vi "GOOP_VI_Provider_Interface.vi"() -> (3 "Interface Table":T1)   [LabVIEW 2014]
uses:
  <resource>/Framework/Providers/API/Provider_Interface.ctl
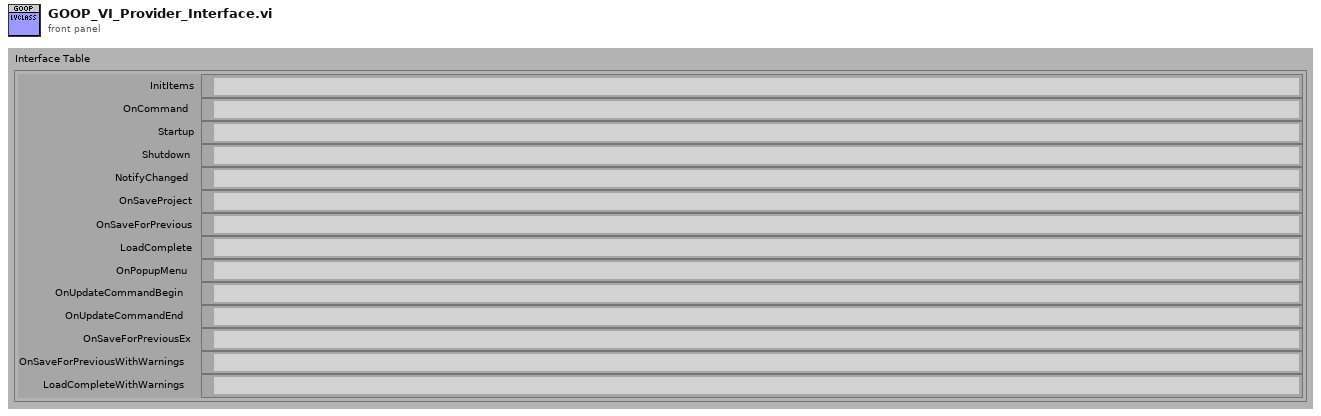
[diagram p1: front panel]
types:
  T1 = typedef "Provider_Interface.ctl" = cluster{"InitItems":path, "OnCommand":path, "Startup":path, "Shutdown":path, "NotifyChanged":path, "OnSaveProject":path, "OnSaveForPrevious":path, "LoadComplete":path, "OnPopupMenu":path, "OnUpdateCommandBegin":path, "OnUpdateCommandEnd":path, "OnSaveForPreviousEx":path, "OnSaveForPreviousWithWarnings":path, "LoadCompleteWithWarnings":path}
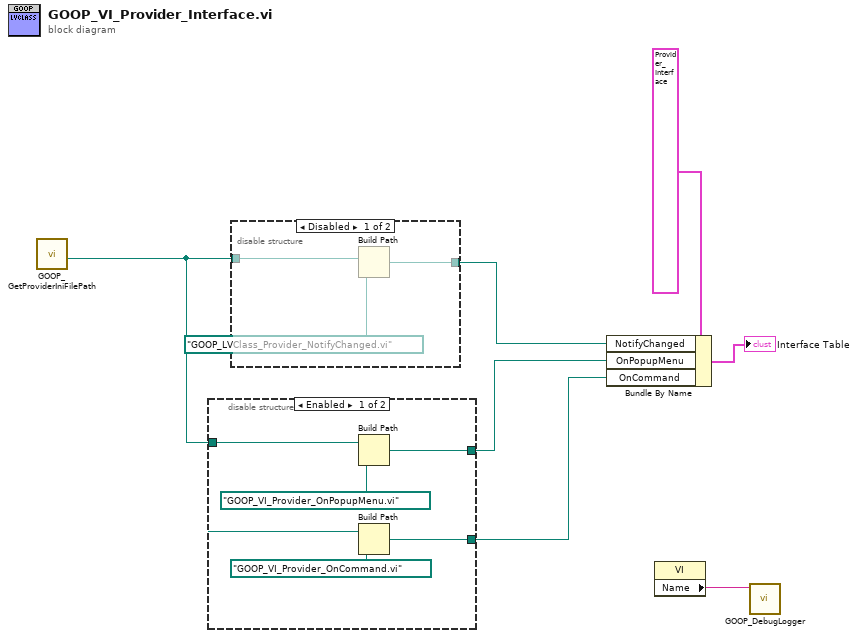
[diagram p0: block diagram]
diagram:
  n1 = call <resource>:"GOOP_GetProviderIniFilePath.vi"() -> ("ProviderMainFolder"=w3:path)  [unwired: 10 in, 1 out]
  n2 = disable-structure shown="Enabled" {
    disable-tunnel: [w11 _] -> w4
    disable-tunnel: w3 -> [w10 _]
    disable-tunnel: [w8 _] -> w2
    frame Enabled {
      n3 = Build Path(base path=w10, name or relative path=path "GOOP_VI_Provider_OnPopupMenu.vi") -> (appended path=w11:path)
      n4 = Build Path(base path=w10, name or relative path=path "GOOP_VI_Provider_OnCommand.vi") -> (appended path=w8:path)
    }
    frame Disabled {
    }
  }
  n5 = disable-structure shown="Disabled" {
    disable-tunnel: [w14 _] -> w5
    disable-tunnel: w3 -> [w13 _]
    frame Disabled {
      n6 = Build Path(base path=w13, name or relative path=path "GOOP_LVClass_Provider_NotifyChanged.vi") -> (appended path=w14:path)
    }
    frame Enabled {
    }
  }
  n7 = Bundle By Name(cluster=T1 {"InitItems"=path "", "OnCommand"=path "", "Startup"=path "", "Shutdown"=path "", "NotifyChanged"=path "", "OnSaveProject"=path "", "OnSaveForPrevious"=path "", "LoadComplete"=path "", "OnPopupMenu"=path "", "OnUpdateCommandBegin"=path "", "OnUpdateCommandEnd"=path "", "OnSaveForPreviousEx"=path "", "OnSaveForPreviousWithWarnings"=path "", "LoadCompleteWithWarnings"=path ""} ("InterfaceTable"), "NotifyChanged"=w5, "OnPopupMenu"=w4, "OnCommand"=w2) -> (→"Interface Table":T1)
  n8 = property class="VI"() -> ("Name"=w1:string)  [unwired: 2 in, 2 out]
  n9 = call <resource>:"GOOP_DebugLogger.vi"("State"=w1) -> ()  [unwired: 8 in, 3 out]
